vi "Set Comment.vi"(8 "error in (no error)":errorcluster, 10 "comment":string, 11 "DOM document in":refnum<k20>) -> (0 "error out":errorcluster, 3 "DOM document out":refnum<k20>)   [LabVIEW 2017, in "Error File Management.lvlib"]
uses:
  Error File Management.lvlib
  <vilib>/xml/Close Reference(Node).vi
  <vilib>/xml/NI_XML.lvlib
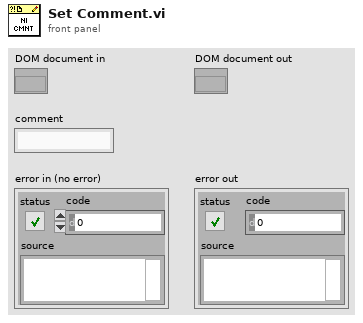
[diagram p1: front panel]
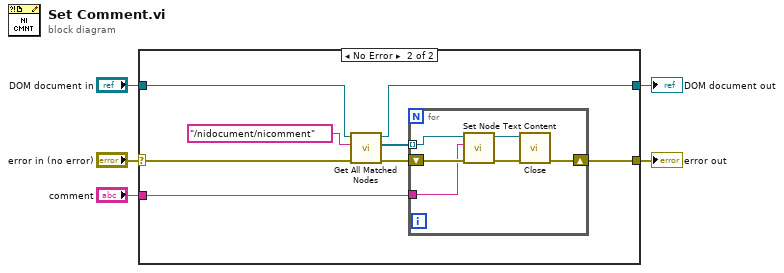
[diagram p0: block diagram]
diagram:
  n1 = case shown="No Error" "error in (no error)" {
    selector: "error in (no error)" -> [w7 w9]
    tunnel: [w6 w15] -> w5
    tunnel: "DOM document in" -> [w6 w14]
    tunnel: [w7 w10] -> w2
    tunnel: "comment" -> [_ w8]
    frame Error {
    }
    frame No Error {
      n2 = call <vilib>:"Get All Matched Nodes.vi"("error in (no error)"=w9, "XPath expression"="/nidocument/nicomment", "node in"=w14) -> ("error out"=w13:errorcluster, "node result array"=w12:refnum<k20>[], "node out"=w15:refnum<k20>)  [unwired: 6 in]
      n3 = for {
        tunnel: w12 -> [w18] mode=indexing
        shift-right: [w21] -> w10
        shift-left: w13 -> [w20]
        tunnel: w8 -> [w16]
        n4 = call "Set Node Text Content.vi"("error in (no error)"=w20, "node text"=w16, "node in"=w18) -> ("error out"=w19:errorcluster, "node out"=w17:refnum<k20>)  [unwired: 7 in]
        n5 = call-poly <vilib>:"Close.vi"("error in (no error)"=w19, "node"=w17) -> ("error out"=w21:errorcluster)  [unwired: 7 out]
      }
    }
  }
  "DOM document out" <- w5
  "error out" <- w2
